vi "VideoCapture Open_FileWithParams.vi"(6 "Params":T2(array[cluster]) {"VideoCaptureProperty" items=["CAP_PROP_POS_MSEC", "CAP_PROP_POS_FRAMES", "CAP_PROP_POS_AVI_RATIO", "CAP_PROP_FRAME_WIDTH", "CAP_PROP_FRAME_HEIGHT", "CAP_PROP_FPS", "CAP_PROP_FOURCC", "CAP_PROP_FRAME_COUNT", "CAP_PROP_FORMAT", "CAP_PROP_MODE", "CAP_PROP_BRIGHTNESS", "CAP_PROP_CONTRAST ", "CAP_PROP_SATURATION", "CAP_PROP_HUE", "CAP_PROP_GAIN", "CAP_PROP_EXPOSURE", "CAP_PROP_CONVERT_RGB", "CAP_PROP_WHITE_BALANCE_BLUE_U", "CAP_PROP_RECTIFICATION", "CAP_PROP_MONOCHROME", "CAP_PROP_SHARPNESS", "CAP_PROP_AUTO_EXPOSURE", "CAP_PROP_GAMMA", "CAP_PROP_TEMPERATURE", "CAP_PROP_TRIGGER ", "CAP_PROP_TRIGGER_DELAY", "CAP_PROP_WHITE_BALANCE_RED_V", "CAP_PROP_ZOOM", "CAP_PROP_FOCUS", "CAP_PROP_GUID", "CAP_PROP_ISO_SPEED", "##", "CAP_PROP_BACKLIGHT", "CAP_PROP_PAN", "CAP_PROP_TILT", "CAP_PROP_ROLL", "CAP_PROP_IRIS", "CAP_PROP_SETTINGS", "CAP_PROP_BUFFERSIZE", "CAP_PROP_AUTOFOCUS", "CAP_PROP_SAR_NUM", "CAP_PROP_SAR_DEN", "CAP_PROP_BACKEND", "CAP_PROP_CHANNEL", "CAP_PROP_AUTO_WB", "CAP_PROP_WB_TEMPERATURE", "CAP_PROP_CODEC_PIXEL_FORMAT", "CAP_PROP_BITRATE ", "CAP_PROP_ORIENTATION_META", "CAP_PROP_ORIENTATION_AUTO", "CAP_PROP_HW_ACCELERATION", "CAP_PROP_HW_DEVICE ", "CAP_PROP_HW_ACCELERATION_USE_OPENCL", "CAP_PROP_OPEN_TIMEOUT_MSEC", "CAP_PROP_READ_TIMEOUT_MSEC", "CAP_PROP_STREAM_OPEN_TIME_USEC", "CAP_PROP_VIDEO_TOTAL_CHANNELS", "CAP_PROP_VIDEO_STREAM", "CAP_PROP_AUDIO_STREAM", "CAP_PROP_AUDIO_POS", "CAP_PROP_AUDIO_SHIFT_NSEC", "CAP_PROP_AUDIO_DATA_DEPTH", "CAP_PROP_AUDIO_SAMPLES_PER_SECOND", "CAP_PROP_AUDIO_BASE_INDEX", "CAP_PROP_AUDIO_TOTAL_CHANNELS", "CAP_PROP_AUDIO_TOTAL_STREAMS", "CAP_PROP_AUDIO_SYNCHRONIZE", "CAP_PROP_LRF_HAS_KEY_FRAME", "CAP_PROP_CODEC_EXTRADATA_INDEX", "CAP_PROP_FRAME_TYPE", "CAP_PROP_N_THREADS", "CAP_PROP_PTS", "CAP_PROP_DTS_DELAY"]}, 8 "error in (no error)":errorcluster, 9 "apiPreference":T3 items=["CAP_ANY"=0, "CAP_VFW/CAP_V4L"=200, "CAP_FIREWIRE"=300, "CAP_QT"=500, "CAP_UNICAP"=600, "CAP_DSHOW"=700, "CAP_PVAPI"=800, "CAP_OPENNI"=900, "CAP_OPENNI_ASUS"=910, "CAP_ANDROID"=1000, "CAP_XIAPI"=1100, "CAP_AVFOUNDATION"=1200, "CAP_GIGANETIX"=1300, "CAP_MSMF"=1400, "CAP_WINRT"=1410, "CAP_INTELPERC/CAP_REALSENSE"=1500, "CAP_OPENNI2"=1600, "CAP_OPENNI2_ASUS"=1610, "CAP_OPENNI2_ASTRA"=1620, "CAP_GPHOTO2"=1700, "CAP_GSTREAMER"=1800, "CAP_FFMPEG"=1900, "CAP_IMAGES"=2000, "CAP_ARAVIS"=2100, "CAP_OPENCV_MJPEG"=2200, "CAP_INTEL_MFX"=2300, "CAP_XINE"=2400, "CAP_UEYE"=2500, "CAP_OBSENSOR"=2600], 10 "Filename":string, 11 "VideoCapture in":refnum<class "VideoCapture.lvclass">) -> (0 "error out":errorcluster, 2 "Success":bool, 3 "VideoCapture out":refnum<class "VideoCapture.lvclass">)   [LabVIEW 2020, in "OpenLvVision_OpenCv.lvlib" / "VideoCapture.lvclass"]
doc: "Opens a video file or a capturing device or an IP video stream for video capturing with API Preference."
uses:
  VideoCapture.lvclass
  C:/Users/lukas/Downloads/OpenLvVision_OpenCv/SourceCode/LabView/OpenLvVision_OpenCv/_LvHelpers/EdvrObject/EdvrObject.lvclass
  TypeDef/VideoCaptureAPIs.ctl
  TypeDef/VideoCaptureProperties.ctl
  _LvHelpers/EdvrObject/EdvrObject.lvclass/EdvrObject.ctl
  OpenLvVision_OpenCv.lvlib
  _LvHelpers/EdvrObject/EdvrObject.lvclass
  Dlls/OlvOpenCvWrapper.dll
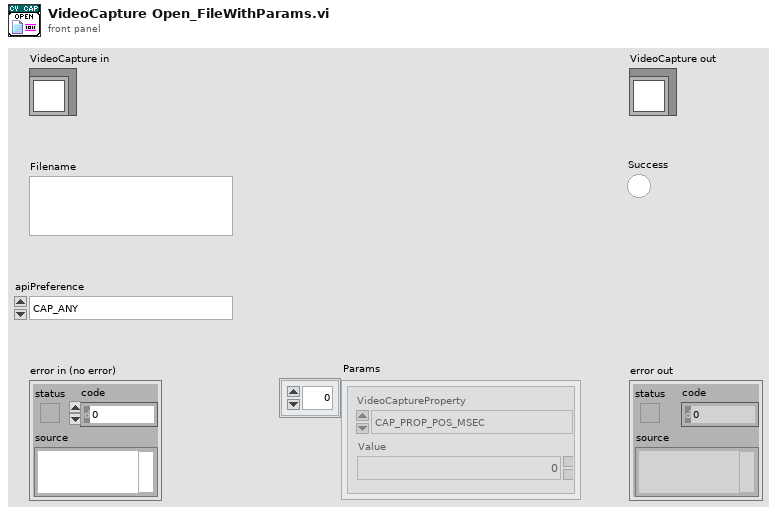
[diagram p1: front panel]
types:
  T1 = typedef "OpenLvVision_OpenCv.lvlib/VideoCaptureProperties.ctl" = i32
  T2 = cluster{"VideoCaptureProperty":T1, "Value":i32}[]
  T3 = typedef "OpenLvVision_OpenCv.lvlib/VideoCaptureAPIs.ctl" = i32
  T4 = typedef "OpenLvVision_OpenCv.lvlib/EdvrObject.lvclass/Edvr.ctl" = refnum<data-value>
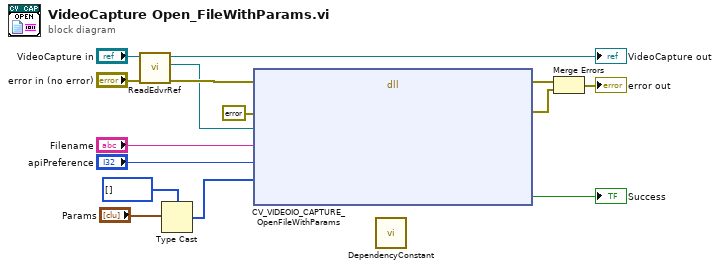
[diagram p0: block diagram]
diagram:
  n1 = call "ReadEdvrRef.vi"("error in (no error)"="error in (no error)", "EdvrObject in"="VideoCapture in") -> ("error out"=w13:errorcluster, "Edvr"=w12:T4, "EdvrObject out"=→"VideoCapture out":refnum<class "VideoCapture.lvclass">)  [unwired: 7 in]
  n2 = Type Cast(type=i32[] [] ("paramsHandle"), x="Params") -> (*(type *) &x=w1:i32[])
  n3 = dll-call lib="C:/Users/lukas/Downloads/OpenLvVision_OpenCv/SourceCode/LabView/OpenLvVision_OpenCv/Dlls/OlvOpenCvWrapper.dll" fn="CV_VIDEOIO_CAPTURE_OpenFileWithParams"(error in=w13, "Error"=errorcluster {"status"=FALSE, "code"=0, "source"=""} ("error out"), "edvrRef"=w12, "filename"="Filename", "apiPreference"="apiPreference", "paramsHandle"=w1) -> (error out=w11:errorcluster, "Error"=w10:errorcluster, "Success"=→"Success":bool)  [unwired: 8 in, 1 out]
  n4 = call "DependencyConstant.vi"() -> ()  [unwired: 12 in]
  n5 = Merge Errors(w11, w10) -> (→"error out":errorcluster)
